vi "MALT Global.vi"() -> ()   [LabVIEW 2018]
panel:
  in  "Parameters":cluster{"Timeout":i32}
  in  "connection ID":refnum<k5>
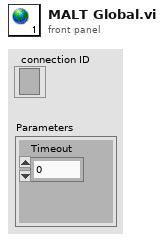
[diagram p1: front panel]
diagram:
